vi "RGB2HSV.vi"(3 "B":u8, 4 "G":u8, 5 "R":u8) -> (0 "V":u8, 1 "S":u8, 2 "H":u8)   [LabVIEW 2021]
doc: "Receives a RGB color and turn it to a HSV format.\nEach color is a U8 data type.\nDesign by Luis Eduardo Rodríguez Ramírez"
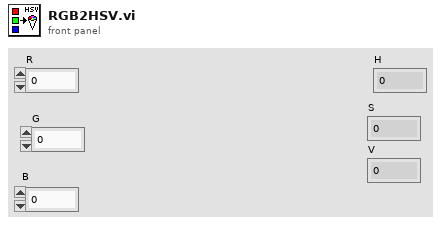
[diagram p1: front panel]
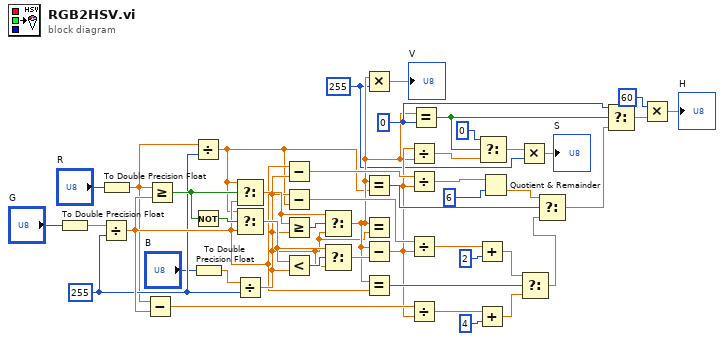
[diagram p0: block diagram]
diagram:
  w8 = u8 255
  w13 = u8 255
  w30 = u8 0
  n1 = To Double Precision Float(number="G") -> (double precision float=w3:dbl)
  n2 = Divide(x=w3, y=w8) -> (x/y=w9:dbl)
  n3 = To Double Precision Float(number="R") -> (double precision float=w5:dbl)
  n4 = Subtract(x=w5, y=w9) -> (x-y=w37:dbl)
  n5 = Greater Or Equal?(x=w5, y=w9) -> (x >= y?=w44:bool)
  n6 = Divide(x=w5, y=w8) -> (x/y=w7:dbl)
  n7 = Not(x=w44) -> (.not. x?=w43:bool)
  n8 = To Double Precision Float(number="B") -> (double precision float=w1:dbl)
  n9 = Select(t=w7, s=w44, f=w9) -> (s? t:f=w45:dbl)
  n10 = Select(t=w7, s=w43, f=w9) -> (s? t:f=w41:dbl)
  n11 = Divide(x=w1, y=w8) -> (x/y=w10:dbl)
  n12 = Subtract(x=w9, y=w10) -> (x-y=w39:dbl)
  n13 = Subtract(x=w10, y=w7) -> (x-y=w38:dbl)
  n14 = Greater Or Equal?(x=w45, y=w10) -> (x >= y?=w46:bool)
  n15 = Less?(x=w41, y=w10) -> (x < y?=w42:bool)
  n16 = Select(t=w45, s=w46, f=w10) -> (s? t:f=w14:dbl)
  n17 = Select(t=w41, s=w42, f=w10) -> (s? t:f=w40:dbl)
  n18 = Multiply(x=w14, y=w13) -> (x*y=→"V":dbl)
  n19 = Equal?(x=w14, y=w7) -> (x = y?=w29:bool)
  n20 = Equal?(x=w14, y=w10) -> ()  [unwired: 1 out]
  n21 = Subtract(x=w14, y=w40) -> (x-y=w18:dbl)
  n22 = Equal?(x=w14, y=w9) -> (x = y?=w25:bool)
  n23 = Divide(x=w18, y=w14) -> (x/y=w17:dbl)
  n24 = Divide(x=w39, y=w18) -> (x/y=w32:dbl)
  n25 = Divide(x=w38, y=w18) -> (x/y=w36:dbl)
  n26 = Divide(x=w37, y=w18) -> (x/y=w33:dbl)
  n27 = Equal?(x=w14, y=w30) -> (x = y?=w20:bool)
  n28 = Add(x=w36, y=u8 2) -> (x+y=w26:dbl)
  n29 = Add(x=w33, y=u8 4) -> (x+y=w24:dbl)
  n30 = Select(t=u8 0, s=w20, f=w17) -> (s? t:f=w16:dbl)
  n31 = Quotient & Remainder(x=w32, y=u8 6) -> (floor(x/y)=w21:dbl)  [unwired: 1 out]
  n32 = Multiply(x=w16, y=w13) -> (x*y=→"S":dbl)
  n33 = Select(t=w26, s=w25, f=w24) -> (s? t:f=w27:dbl)
  n34 = Select(t=w21, s=w29, f=w27) -> (s? t:f=w28:dbl)
  n35 = Select(t=w30, s=w20, f=w28) -> (s? t:f=w23:dbl)
  n36 = Multiply(x=u8 60, y=w23) -> (x*y=→"H":dbl)
